vi "Get Server Stop UE.vi"(11 "OOP Server in":refnum<class "MeasurementService_Template.lvclass">) -> (2 "Server Stop":refnum<user-event>, 3 "OOP Server out":refnum<class "MeasurementService_Template.lvclass">)   [LabVIEW 2020, in "LineRegulation.lvlib" / "MeasurementService_Template.lvclass"]
uses:
  MeasurementService_Template.lvclass
  MeasurementService_Template.lvclass/MeasurementService_Template.ctl
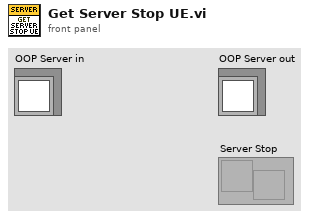
[diagram p1: front panel]
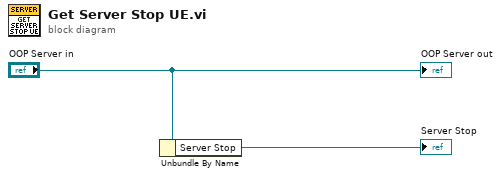
[diagram p0: block diagram]
diagram:
  n1 = Unbundle By Name("OOP Server in") -> ("Server Stop"=→"Server Stop":refnum<user-event>)
  "OOP Server out" <- "OOP Server in"
